vi "getAUX.vi"(8 "error in (no error)":errorcluster, 10 "Channel":i32=1 min=1 max=16, 11 "Instrument.LockinAPI in":refnum<class "Instrument.LockinAPI.lvclass">) -> (0 "error out":errorcluster, 2 "AUX (V)":dbl, 3 "Instrument.LockinAPI out":refnum<class "Instrument.LockinAPI.lvclass">)   [LabVIEW 2019, in "Instrument.LockinAPI.lvclass"]
doc: "API to get value of any auxiliary channels\n\nIf address=\"\", this API reads from localhost\nIf address is remote lockin, you need to add this computer to allowed whitelist on the lockin computer you are trying to access."
uses:
  Instrument.LockinAPI.lvclass
  Typedefs/LockinAPI.Commands--Enum.ctl
  d4117681-07e7-4ebe-9255-c065752609da.vi
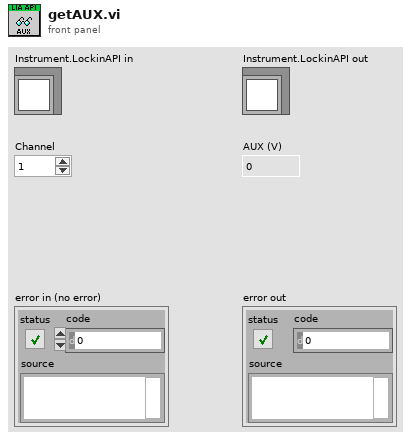
[diagram p1: front panel]
types:
  T1 = typedef "Instrument.LockinAPI.lvclass/LockinAPI.commands--Enum.ctl" = enum16{"setAI", "setAO", "setAO_Amplitude", "setAO_DC", "setAO_Frequency", "setAO_Phase", "setAO_Function", "setAO_I+", "setREF", "setREF_Frequency", "setREF_Phase", "setREF_TC", "setREF_Roll-Off", "setDAQ", "setSampling", "setOffset", "setState", "getState", "getAO", "getAI", "getResults", "getSampling", "getAOconfig", "getREFconfig", "setInputGain", "setOutputGain", "getInputGain", "getOutputGain", "setSamplingMode", "getSamplingMode", "setSweep", "setSweepTime", "setSweepTable", "getStatus", "getSweepResults", "getSweepWaveforms", "startSweep", "stopSweep", "setAUX", "getAUX"}
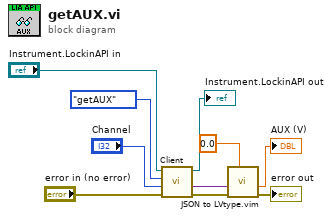
[diagram p0: block diagram]
diagram:
  n1 = call-dynamic "Client.vi"("error in (no error)"="error in (no error)", "Data in"="Channel", "Command in"=LockinAPI.commands--Enum."getAUX" ("Command"), "Instrument in"="Instrument.LockinAPI in") -> ("error out"=w5:errorcluster, "Data out"=w3:variant, "Instrument out"=→"Instrument.LockinAPI out":refnum<class "Instrument.LockinAPI.lvclass">)  [unwired: 4 in, 1 out]
  n2 = call "JSON to LVtype.vim"("type"=0.0 ("AUX (V)"), "error in (no error)"=w5, "JSON Data in"=w3) -> ("error out"=→"error out":errorcluster, "Data out"=→"AUX (V)":dbl)  [unwired: 7 in]
